vi "testConvertToObjectMapAndSetToParameter.vi"() -> ()   [LabVIEW 2017]
uses:
  Common/ObjectMap/LVPortObjectMapNamepathData.ctl
  Common/ObjectMap/LVPortObjectMapDataTypeEnum.ctl
  Common/ObjectMap/LVPortObjectMapContainerTypeEnum.ctl
  Common/ObjectMap/LVPortObjectMapDefaultIDsEnum.ctl
panel:
  out "Temp Value ID":i32
  out "Matlab Param Data":T1[](array[typedef])
  in  "SomeVal":T4
  out "pID":string
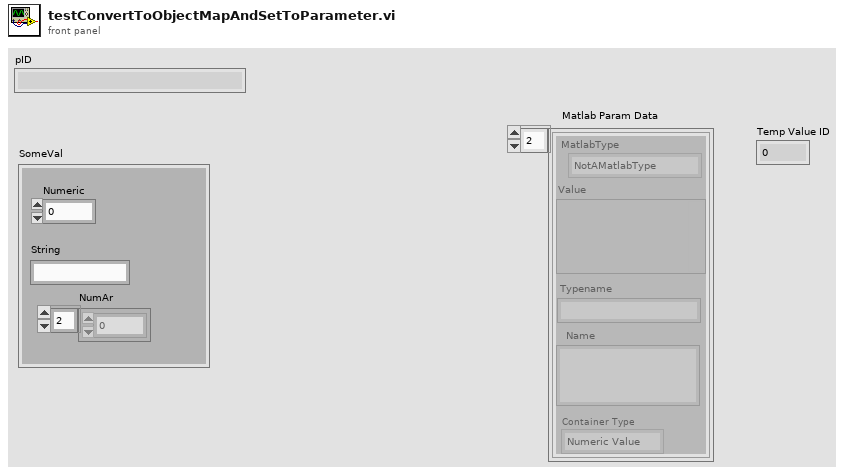
[diagram p1: front panel]
types:
  T1 = typedef "LVPortObjectMapNamepathData.ctl" = cluster{"MatlabType":T2, "Value":variant, "Name":string, "Typename":string, "Container Type":T3}
  T2 = typedef "LVPortObjectMapDataTypeEnum.ctl" = enum16{"NotAMatlabType", "Real", "Complex", "String", "Boolean"}
  T3 = typedef "LVPortObjectMapContainerTypeEnum.ctl" = enum16{"Numeric Value", "Numeric Array", "Waveform"}
  T4 = cluster{"Numeric":dbl, "String":string, "NumAr":dbl[]}
  T5 = typedef "LVPortObjectMapDefaultIDsEnum.ctl" = i32
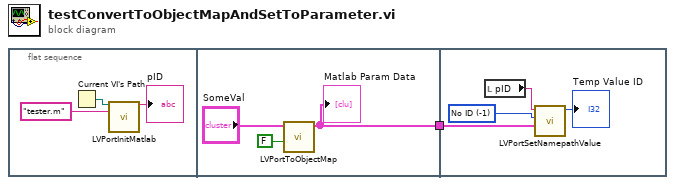
[diagram p0: block diagram]
diagram:
  n1 = flat-sequence {
    tunnel: [w6] -> w1
    tunnel: w1 -> [w9]
    frame #0 {
      n2 = Current VI's Path() -> (path=w4:path)
      n3 = call "LVPortInitMatlab.vi"("Working directory or VI Path"=w4, "Code file name"="tester.m") -> ("ID"=→"pID":string)  [unwired: 12 in, 1 out]
    }
    frame #1 {
      n4 = call "LVPortToObjectMap.vi"("Skip Parent Name"=FALSE ("IgnoreContainerName"), "Value"="SomeVal") -> ("Object map"=w6:T1[])  [unwired: 9 in]
      "Matlab Param Data" <- w6
    }
    frame #2 {
      w10 = T5 -1 items=["No ID"=-1, "Port Object"=-2] ("Default IDs")
      n5 = local read "pID"() -> (w11:string)
      n6 = call "LVPortSetNamepathValue.vi"("ObjectMap"=w9, "Object ID"=w10, "pID"=w11) -> ("Object ID (Validated)"=→"Temp Value ID":i32)  [unwired: 6 in, 2 out]
    }
  }
